vi "Create_Folder (SubVI).vi"(8 "error in":errorcluster, 9 "Name":string, 10 "Three position":T1, 11 "Path":path) -> (0 "error out":errorcluster, 3 "created path":path)   [LabVIEW 2011]
uses:
  Ctl/EnumThreePosition.ctl
  <vilib>/regexp/Match Regular Expression.xnode
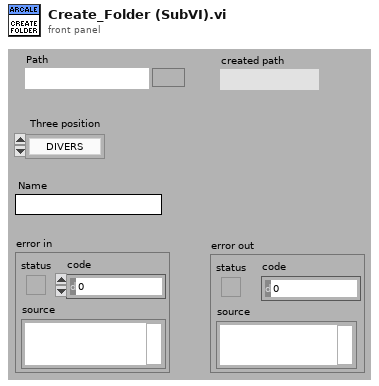
[diagram p1: front panel]
types:
  T1 = typedef "EnumThreePosition.ctl" = enum16{"DIVERS", "MAIN", "SPLASH SCREEN", "HMI", "EVENTS", "SCREENS", "CONFIG", "TOOLS", "ERRORS", "PROCESS"}
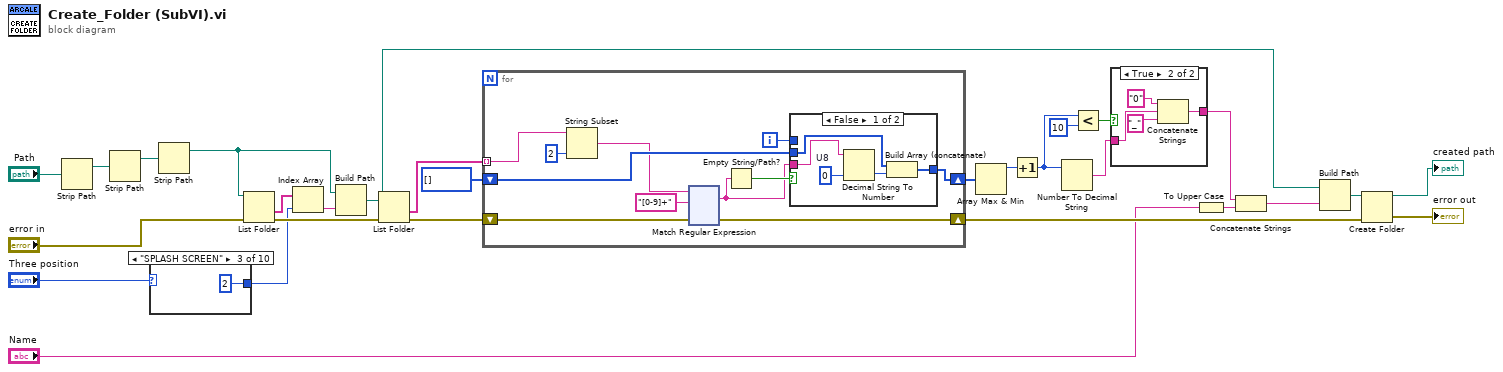
[diagram p0: block diagram]
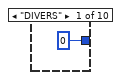
[diagram p2: hidden frame]
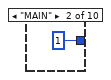
[diagram p3: hidden frame]
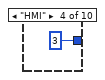
[diagram p4: hidden frame]
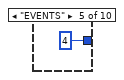
[diagram p5: hidden frame]
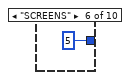
[diagram p6: hidden frame]
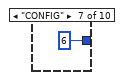
[diagram p7: hidden frame]
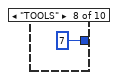
[diagram p8: hidden frame]
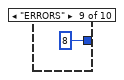
[diagram p9: hidden frame]
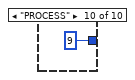
[diagram p10: hidden frame]
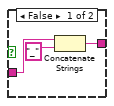
[diagram p11: hidden frame]
diagram:
  n1 = Strip Path(path="Path") -> (stripped path=w10:path)  [unwired: 1 out]
  n2 = Strip Path(path=w10) -> (stripped path=w23:path)  [unwired: 1 out]
  n3 = case shown="\"SPLASH SCREEN\"" "Three position" {
    tunnel: [0 1 2 3 4 5 6 7 8 9] -> w6
    frame "DIVERS" {
    }
    frame "MAIN" {
    }
    frame "SPLASH SCREEN" {
    }
    frame "HMI" {
    }
    frame "EVENTS" {
    }
    frame "SCREENS" {
    }
    frame "CONFIG" {
    }
    frame "TOOLS" {
    }
    frame "ERRORS" {
    }
    frame "PROCESS" {
    }
  }
  n4 = Strip Path(path=w23) -> (stripped path=w7:path)  [unwired: 1 out]
  n5 = List Folder(path=w7, error in="error in") -> (folder names=w21:string[], error out=w24:errorcluster)  [unwired: 2 in, 2 out]
  n6 = Index Array(array=w21, index=w6) -> (element=w22:string)
  n7 = Build Path(base path=w7, name or relative path=w22) -> (appended path=w5:path)
  n8 = List Folder(path=w5, error in=w24) -> (folder names=w4:string[], error out=w26:errorcluster)  [unwired: 2 in, 2 out]
  n9 = for {
    tunnel: w4 -> [w40] mode=indexing
    shift-right: [w47] -> w27
    shift-left: w26 -> [w48]
    shift-right: [w43] -> w2
    shift-left: u8[] [] -> [w42]
    i -> [w44]
    n10 = String Subset(string=w40, length (rest)=2 ("length (rest)")) -> (substring=w39:string)  [unwired: 1 in]
    n11 = xnode "Match Regular Expression"("input string"=w39, "regular expression"="[0-9]+", "error in"=w48) -> ("whole match"=w45:string, "error out"=w47:errorcluster)  [unwired: 3 in, 3 out]
    n12 = Empty String/Path?(string/path=w45) -> (empty?=w46:bool)
    n13 = case shown="False" w46 {
      tunnel: w45 -> [w53 _]
      tunnel: w44 -> [_ _]
      tunnel: [w51 w55] -> w43
      tunnel: w42 -> [w50 w55]
      frame False {
        w54 = u8 0  # U8
        n14 = Decimal String To Number(string=w53, default (0L)=w54) -> (number=w52:u8)  [unwired: 1 in, 1 out]
        n15 = Build Array (concatenate)(w50, w52) -> (w51:u8[])
      }
      frame True {
      }
    }
  }
  n16 = Array Max & Min(array=w2) -> (max value=w11:u8)  [unwired: 3 out]
  n17 = Increment(x=w11) -> (x+1=w14:u8)
  n18 = Number To Decimal String(number=w14) -> (decimal integer string=w15:string)  [unwired: 1 in]
  n19 = Less?(x=w14, y=u8 10) -> (x < y?=w13:bool)
  n20 = case shown="True" w13 {
    tunnel: w15 -> [w169 w173]
    tunnel: [w167 w170] -> w16
    frame False {
      n21 = Concatenate Strings(w169, "_" ("string")) -> (w167:string)
    }
    frame True {
      n22 = Concatenate Strings("0" ("string"), w173, "_" ("string")) -> (w170:string)
    }
  }
  n23 = To Upper Case(1:"Name") -> (0:w17:string)
  n24 = Concatenate Strings(w16, w17) -> (w18:string)
  n25 = Build Path(base path=w5, name or relative path=w18) -> (appended path=w19:path)
  n26 = Create Folder(path (use dialog)=w19, error in=w27) -> (created path=→"created path":path, error out=→"error out":errorcluster)  [unwired: 1 in, 1 out]
